vi "Example - Cluster Standard retrieve rulers.vi"() -> ()   [LabVIEW 2017]
uses:
  91606217-0aa9-4d15-96b7-8b297c548ea6.vi
  1666e5c6-ebfe-49ef-8ce9-ca26aba7fc85.vi
  0581107d-8152-4841-aa39-46f148f37cd2.vi
  8f60ddcf-0cb1-4fc8-acc6-41852b9c13b8.vi
  2fe488ef-b7bb-44d0-a25d-5ffd90c1f184.vi
  a9cae98a-f907-4981-8728-e4dab4e61435.vi
  6d8c267f-2772-4021-96a0-a112b934f822.vi
  af806db9-11e8-4920-a3d8-4dc6becce253.vi
  32ee3063-d89e-4a28-9b2b-c8f76bed8ce1.vi
  9953fe41-aef1-4428-9d31-84e750963704.vi
  19c0801d-dea2-467e-8f01-f7ea4b210c2b.vi
  e305bcdb-14a9-4ef8-b0a2-667a5c074ea4.vi
  API-String-Arugments-Support/_Support/Convert API String Arguments to Data(variant).vi
panel:
  out "output cluster 12":T1={"String"="a:1;xxx.yyy.c:2;d:3;zzz.d:4", "Reference Cluster"={"a"="", "xxx"={"b"="", "c"="", "yyy"={"d"="", "c"=""}}, "zzz"={"c"="", "d"=""}}, "Retrieved Cluster"={"a"="1", "xxx"={"b"="", "c"="", "yyy"={"d"="3", "c"="2"}}, "zzz"={"c"="", "d"="4"}}}
  out "output cluster 11":T1={"String"="a:1;yyy.c:2;d:3;zzz.d:4", "Reference Cluster"={"a"="", "xxx"={"b"="", "c"="", "yyy"={"d"="", "c"=""}}, "zzz"={"c"="", "d"=""}}, "Retrieved Cluster"={"a"="1", "xxx"={"b"="", "c"="", "yyy"={"d"="3", "c"="2"}}, "zzz"={"c"="", "d"="4"}}}
  out "output cluster 10":T1={"String"="a:1;c:2;d:3;zzz.d:4", "Reference Cluster"={"a"="", "xxx"={"b"="", "c"="", "yyy"={"d"="", "c"=""}}, "zzz"={"c"="", "d"=""}}, "Retrieved Cluster"={"a"="1", "xxx"={"b"="", "c"="2", "yyy"={"d"="3", "c"=""}}, "zzz"={"c"="", "d"="4"}}}
  out "output cluster 9":T2={"String"="[a,b,c];Name:xxx;xxx:1", "Reference Cluster"={"Child"=[], "Name"="abc", "Bool"=FALSE}, "Data"={"Child"=["a", "b", "c"], "Name"="Name:xxx", "Bool"=TRUE}}
  out "output cluster 8":T2={"String"="[a,b,c];234;1", "Reference Cluster"={"Child"=[], "Name"="abc", "Bool"=FALSE}, "Data"={"Child"=["a", "b", "c"], "Name"="234", "Bool"=TRUE}}
  out "output cluster 7":T2={"String"="Name:xyz", "Reference Cluster"={"Child"=[], "Name"="abc", "Bool"=FALSE}, "Data"={"Child"=[], "Name"="xyz", "Bool"=FALSE}}
  out "output cluster 6":T2={"String"="[a,b,c];234", "Reference Cluster"={"Child"=[], "Name"="abc", "Bool"=FALSE}, "Data"={"Child"=["a", "b", "c"], "Name"="234", "Bool"=FALSE}}
  out "output cluster 5":T2={"String"="[a,b,c];234;on", "Reference Cluster"={"Child"=[], "Name"="abc", "Bool"=FALSE}, "Data"={"Child"=["a", "b", "c"], "Name"="234", "Bool"=TRUE}}
  out "output cluster 4":T2={"String"="xyz", "Reference Cluster"={"Child"=[], "Name"="abc", "Bool"=FALSE}, "Data"={"Child"=["xyz"], "Name"="abc", "Bool"=FALSE}}
  out "output cluster 3":T3={"Input String"="xyz", "Reference Cluster"={"Name"="abc", "Child"={"Name"="ddd"}, "Bool"=FALSE}, "Retrieved Cluster"={"Name"="xyz", "Child"={"Name"="ddd"}, "Bool"=FALSE}}
  out "output cluster 2":T3={"Input String"="Name:xxx", "Reference Cluster"={"Name"="abc", "Child"={"Name"="ddd"}, "Bool"=FALSE}, "Retrieved Cluster"={"Name"="xxx", "Child"={"Name"="ddd"}, "Bool"=FALSE}}
  out "output cluster 1":T3={"Input String"="", "Reference Cluster"={"Name"="abc", "Child"={"Name"="ddd"}, "Bool"=FALSE}, "Retrieved Cluster"={"Name"="abc", "Child"={"Name"="ddd"}, "Bool"=FALSE}}
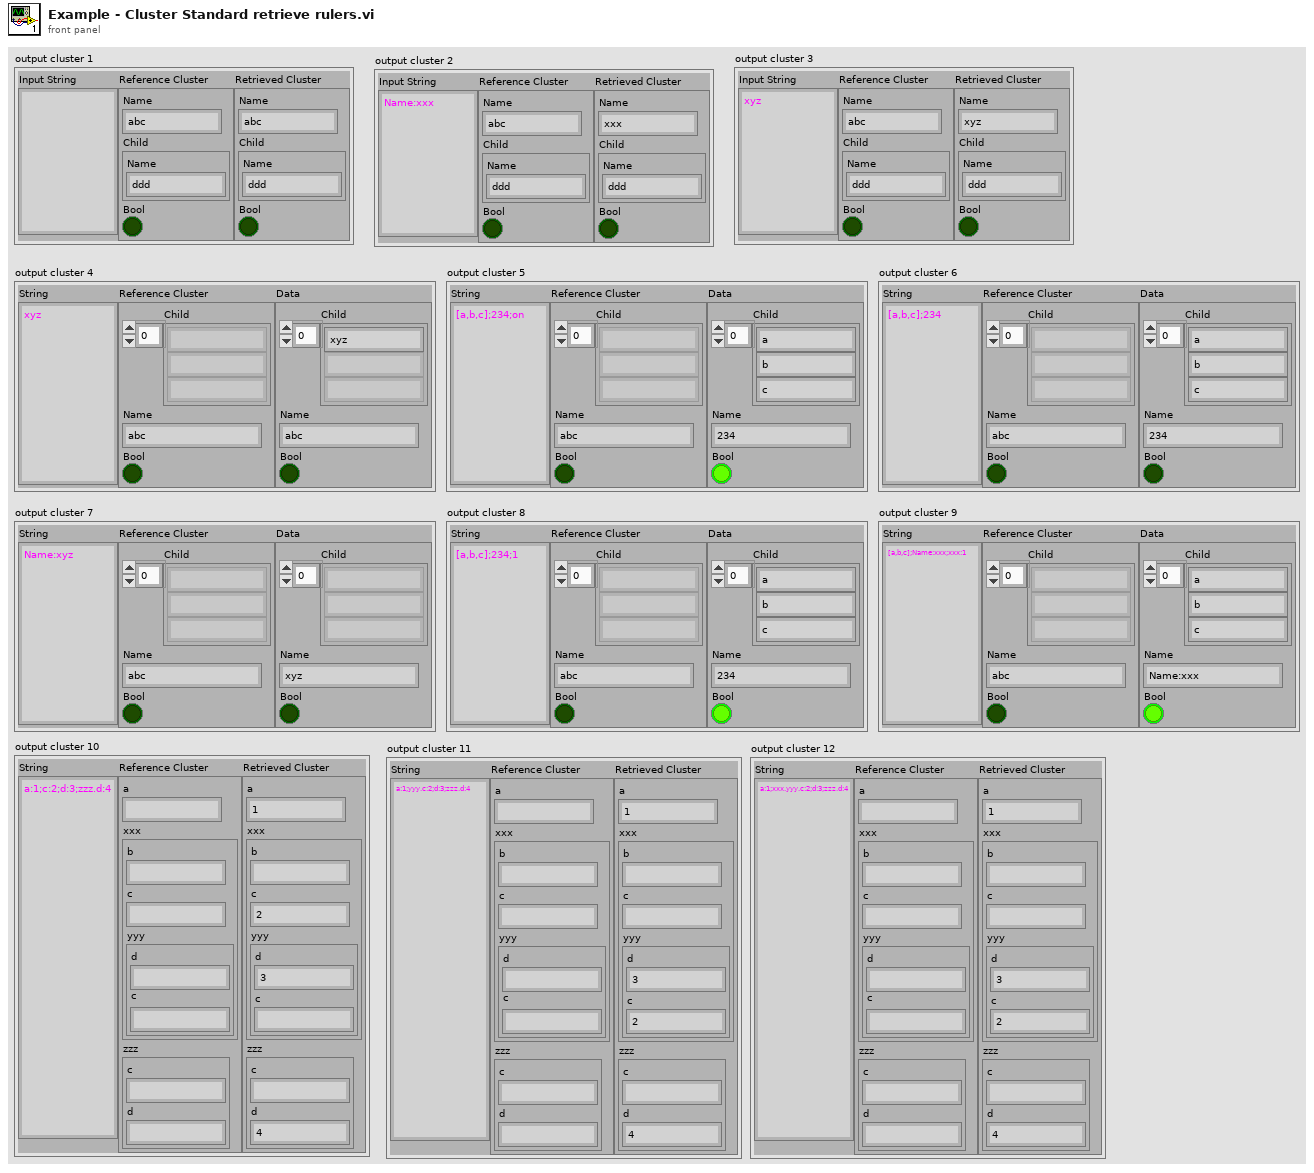
[diagram p1: front panel]
types:
  T1 = cluster{"String":string, "Reference Cluster":cluster{"a":string, "xxx":cluster{"b":string, "c":string, "yyy":cluster{"d":string, "c":string}}, "zzz":cluster{"c":string, "d":string}}, "Retrieved Cluster":cluster{"a":string, "xxx":cluster{"b":string, "c":string, "yyy":cluster{"d":string, "c":string}}, "zzz":cluster{"c":string, "d":string}}}
  T2 = cluster{"String":string, "Reference Cluster":cluster{"Child":string[], "Name":string, "Bool":bool}, "Data":cluster{"Child":string[], "Name":string, "Bool":bool}}
  T3 = cluster{"Input String":string, "Reference Cluster":cluster{"Name":string, "Child":cluster{"Name":string}, "Bool":bool}, "Retrieved Cluster":cluster{"Name":string, "Child":cluster{"Name":string}, "Bool":bool}}
  T4 = cluster{"a":string, "xxx":cluster{"b":string, "c":string, "yyy":cluster{"d":string, "c":string}}, "zzz":cluster{"c":string, "d":string}}
  T5 = cluster{"Name":string, "Child":cluster{"Name":string}, "Bool":bool}
  T6 = cluster{"Child":string[], "Name":string, "Bool":bool}
  T7 = cluster{"String":string, "Reference Cluster":cluster{"Name":string, "Child":cluster{"Name":string}, "Bool":bool}, "Data":cluster{"Name":string, "Child":cluster{"Name":string}, "Bool":bool}}
  T8 = cluster{"String":string, "Reference Cluster 2":cluster{"Child":string[], "Name":string, "Bool":bool}, "Data":cluster{"Child":string[], "Name":string, "Bool":bool}}
  T9 = cluster{"String":string, "Reference Cluster 3":cluster{"a":string, "xxx":cluster{"b":string, "c":string, "yyy":cluster{"d":string, "c":string}}, "zzz":cluster{"c":string, "d":string}}, "Data":cluster{"a":string, "xxx":cluster{"b":string, "c":string, "yyy":cluster{"d":string, "c":string}}, "zzz":cluster{"c":string, "d":string}}}
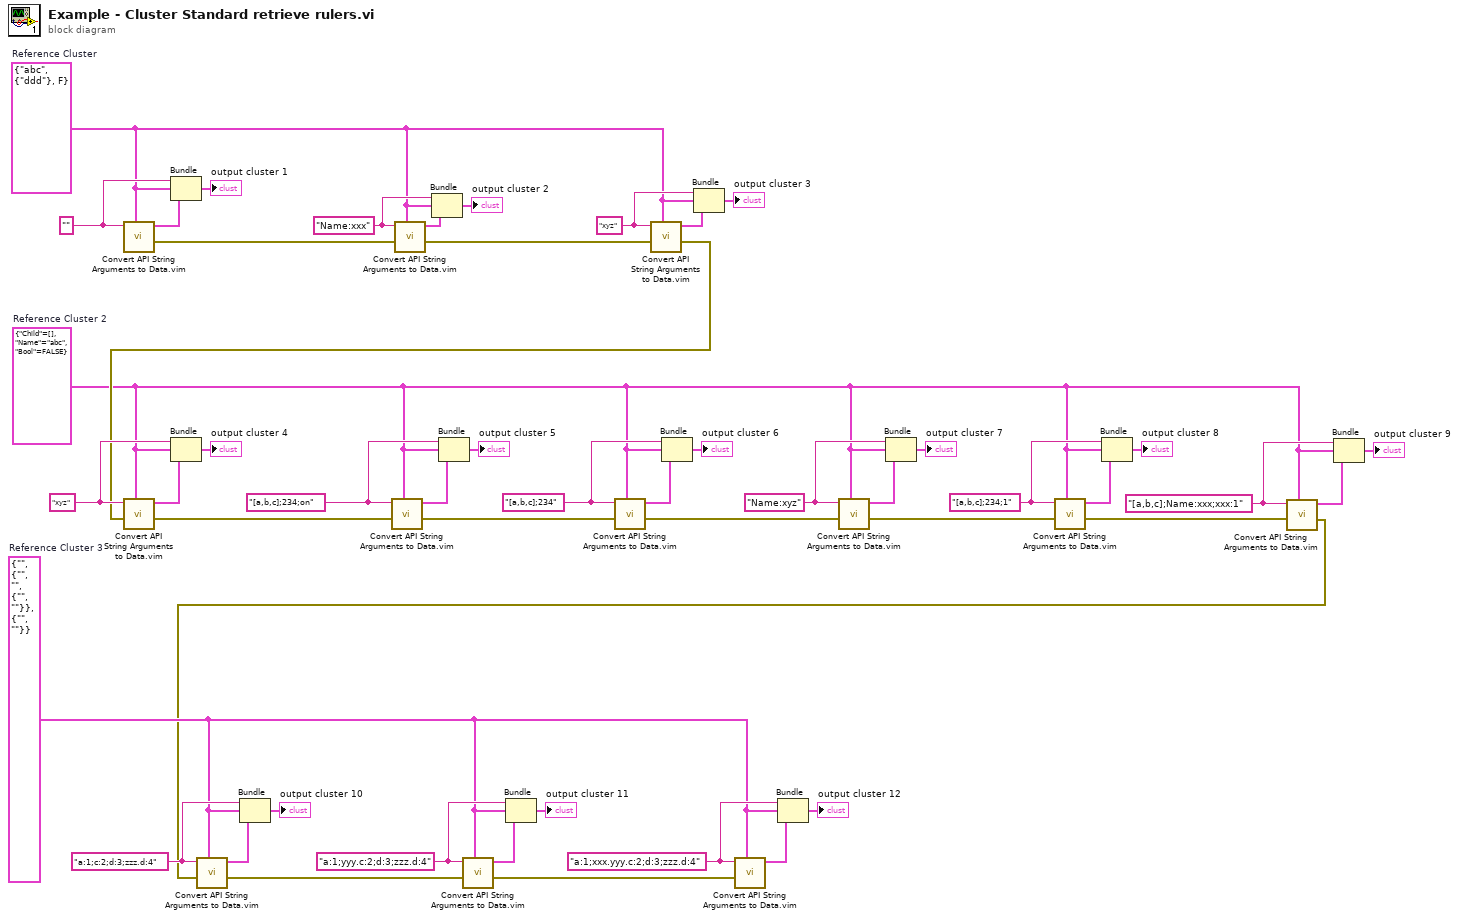
[diagram p0: block diagram]
diagram:
  w6 = "a:1;xxx.yyy.c:2;d:3;zzz.d:4" ("String")
  w8 = "a:1;yyy.c:2;d:3;zzz.d:4" ("String")
  w16 = "[a,b,c];Name:xxx;xxx:1" ("String")
  w22 = "[a,b,c];234;1" ("String")
  w23 = "Name:xyz" ("String")
  w45 = "Name:xxx" ("String")
  w13 = "a:1;c:2;d:3;zzz.d:4" ("String")
  w2 = T4 {"a"="", "xxx"={"b"="", "c"="", "yyy"={"d"="", "c"=""}}, "zzz"={"c"="", "d"=""}}  # Reference Cluster 3
  w29 = "[a,b,c];234" ("String")
  w33 = "[a,b,c];234;on" ("String")
  w50 = "" ("String")
  w40 = T5 {"Name"="abc", "Child"={"Name"="ddd"}, "Bool"=FALSE}  # Reference Cluster
  w38 = "xyz" ("String")
  w15 = T6 {"Child"=[], "Name"="abc", "Bool"=FALSE}  # Reference Cluster 2
  w41 = "xyz" ("String")
  n1 = call "Convert API String Arguments to Data.vim"("Type"=w40, "String"=w50) -> ("error"=w47:errorcluster, "Data"=w49:T5)  [unwired: 6 in]
  n2 = Bundle("String"=w50, "Reference Cluster"=w40, "Data"=w49) -> (→"output cluster 1":T7)  [unwired: 1 in]
  n3 = call "Convert API String Arguments to Data.vim"("Type"=w40, "error in (no error)"=w47, "String"=w45) -> ("error"=w43:errorcluster, "Data"=w44:T5)  [unwired: 5 in]
  n4 = Bundle("String"=w45, "Reference Cluster"=w40, "Data"=w44) -> (→"output cluster 2":T7)  [unwired: 1 in]
  n5 = call "Convert API String Arguments to Data.vim"("Type"=w40, "error in (no error)"=w43, "String"=w41) -> ("error"=w28:errorcluster, "Data"=w39:T5)  [unwired: 5 in]
  n6 = call "Convert API String Arguments to Data.vim"("Type"=w15, "error in (no error)"=w28, "String"=w38) -> ("error"=w27:errorcluster, "Data"=w37:T6)  [unwired: 5 in]
  n7 = Bundle("String"=w38, "Reference Cluster 2"=w15, "Data"=w37) -> (→"output cluster 4":T8)  [unwired: 1 in]
  n8 = call "Convert API String Arguments to Data.vim"("Type"=w15, "error in (no error)"=w27, "String"=w33) -> ("error"=w30:errorcluster, "Data"=w35:T6)  [unwired: 5 in]
  n9 = Bundle("String"=w33, "Reference Cluster 2"=w15, "Data"=w35) -> (→"output cluster 5":T8)  [unwired: 1 in]
  n10 = call "Convert API String Arguments to Data.vim"("Type"=w15, "error in (no error)"=w30, "String"=w29) -> ("error"=w24:errorcluster, "Data"=w31:T6)  [unwired: 5 in]
  n11 = Bundle("String"=w29, "Reference Cluster 2"=w15, "Data"=w31) -> (→"output cluster 6":T8)  [unwired: 1 in]
  n12 = Bundle("String"=w41, "Reference Cluster"=w40, "Data"=w39) -> (→"output cluster 3":T7)  [unwired: 1 in]
  n13 = call "Convert API String Arguments to Data.vim"("Type"=w15, "error in (no error)"=w24, "String"=w23) -> ("error"=w19:errorcluster, "Data"=w26:T6)  [unwired: 5 in]
  n14 = Bundle("String"=w23, "Reference Cluster 2"=w15, "Data"=w26) -> (→"output cluster 7":T8)  [unwired: 1 in]
  n15 = call "Convert API String Arguments to Data.vim"("Type"=w15, "error in (no error)"=w19, "String"=w22) -> ("error"=w14:errorcluster, "Data"=w20:T6)  [unwired: 5 in]
  n16 = Bundle("String"=w22, "Reference Cluster 2"=w15, "Data"=w20) -> (→"output cluster 8":T8)  [unwired: 1 in]
  n17 = call "Convert API String Arguments to Data.vim"("Type"=w15, "error in (no error)"=w14, "String"=w16) -> ("error"=w1:errorcluster, "Data"=w18:T6)  [unwired: 5 in]
  n18 = call "Convert API String Arguments to Data.vim"("Type"=w2, "error in (no error)"=w1, "String"=w13) -> ("error"=w7:errorcluster, "Data"=w12:T4)  [unwired: 5 in]
  n19 = Bundle("String"=w13, "Reference Cluster 3"=w2, "Data"=w12) -> (→"output cluster 10":T9)  [unwired: 1 in]
  n20 = call "Convert API String Arguments to Data.vim"("Type"=w2, "error in (no error)"=w7, "String"=w8) -> ("error"=w3:errorcluster, "Data"=w9:T4)  [unwired: 5 in]
  n21 = Bundle("String"=w8, "Reference Cluster 3"=w2, "Data"=w9) -> (→"output cluster 11":T9)  [unwired: 1 in]
  n22 = call "Convert API String Arguments to Data.vim"("Type"=w2, "error in (no error)"=w3, "String"=w6) -> ("Data"=w5:T4)  [unwired: 5 in, 1 out]
  n23 = Bundle("String"=w6, "Reference Cluster 3"=w2, "Data"=w5) -> (→"output cluster 12":T9)  [unwired: 1 in]
  n24 = Bundle("String"=w16, "Reference Cluster 2"=w15, "Data"=w18) -> (→"output cluster 9":T8)  [unwired: 1 in]
